vi "Initialize.vi"(11 "Device Reference":T40 format="%.0x") -> (0 "error out":errorcluster, 3 "RT Data":T1 {"Compiled Data"."1.1 APUs"."shared settings"."cycle start" format="%#.15g"; "Compiled Data"."1.0 APUs"."shared settings"."cycle start" format="%#.15g"})   [LabVIEW 2013, in "Engine Simulation Toolkit Engine.lvlib"]
uses:
  Engine Simulation Toolkit Engine.lvlib
  <vilib>/NI Veristand/Custom Device API/Custom Device Item Ref.ctl
  RT Data.ctl
  Shared/Compiled Data.ctl
  Shared/Engine Init Data.ctl
  Shared/1.0 APU Engine Data.ctl
  Shared/1.0 APU Engine FIFO Idxs.ctl
  Shared/Engine Status Data.ctl
  Shared/1.0 Analog Replay Engine Data.ctl
  Shared/1.0 Analog Replay FIFO Idxs.ctl
  Shared/1.0 Digital Pattern Gen Engine Data.ctl
  Shared/1.0 Digital Pattern Gen FIFO Idxs.ctl
  Shared/1.0 Event Timing Capture Engine Data.ctl
  Shared/1.0 Event Timing Capture FIFO Idxs.ctl
  Shared/1.0 Event Timing Measure Engine Data.ctl
  Shared/1.0 Event Timing Measure FIFO Idxs.ctl
  Shared/1.0 Knock Sensor Engine Data.ctl
  Shared/1.0 Knock Sensor FIFO Idxs.ctl
  Shared/1.0 Knock Cylinder Engine Data.ctl
  Shared/1.0 Knock Cylinder FIFO Idxs.ctl
  Shared/1.0 Directional Speed Engine Data.ctl
  Shared/1.0 Directional Speed FIFO Idxs.ctl
  Shared/1.1 APU Engine Data.ctl
  Shared/1.1 Event Timing Measure Engine Data.ctl
  Shared/1.3 Digital Pattern Gen Engine Data.ctl
  Shared/1.3 Digital Pattern Gen FIFO Idxs.ctl
  Shared/Bitfile EST Version.ctl
  Shared/1.3 APU Engine Data.ctl
  FPGA Refs.ctl
  APU 1.0 Run Refs.ctl
  APU 1.0 Output Ref.ctl
  APU 1.0 Input Ref.ctl
  Analog Replay 1.0 Input Ref.ctl
  Digital Pattern Gen 1.0 Input Ref.ctl
  Event Timing Capture 1.0 Output Ref.ctl
  Event Timing Measure 1.0 Output Ref.ctl
  Knock Cylinder 1.0 Input Ref.ctl
  Knock Sensor 1.0 Input Ref.ctl
  Directional Speed 1.0 Input Ref.ctl
  Digital Pattern Gen 1.3 Run Refs.ctl
  Digital Pattern Gen 1.3 Settings Ref.ctl
  Shared/Properties.vi
  <vilib>/NI Veristand/Custom Device API/Get Item Property (Variant).vi
  <vilib>/NI Veristand/Custom Device API/Custom Device API.lvlib
  Shared/Engine Simulation Toolkit Shared.lvlib
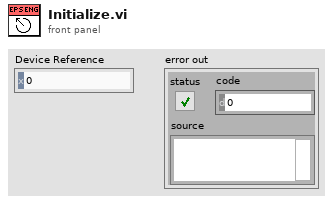
[diagram p1: front panel]
types:
  T1 = typedef "Engine Simulation Toolkit Engine.lvlib/RT Data.ctl" = cluster{"Compiled Data":T2, "FPGA Refs":T27}
  T2 = typedef "Engine Simulation Toolkit Shared.lvlib/Compiled Data.ctl" = cluster{"Init":T3, "1.0 APUs":T4[], "Status":T6, "DevOutFIFO":refnum<k33>, "DevInFIFO":refnum<k33>, "Device Inputs":dbl[], "Device Outputs":dbl[], "Last Device Inputs":dbl[], "1.0 Analog Replays":T7[], "Unused Analog Replays":string[], "1.0 Digital Pattern Gens":T9[], "Unused Digital Pattern Gens":string[], "1.0 Event Captures":T11[], "1.0 Event Measures":T13[], "1.0 Knock Sensors":T15[], "1.0 Knock Cylinders":T17[], "1.0 Directional Speed":T19[], "Unused Directional Sensors":string[], "1.1 APUs":T21[], "1.1 Event Measures":T22[], "1.3 Digital Pattern Gens":T23[], "Bitfile EST Version":T25, "1.3 APUs":T26[]}
  T3 = typedef "Engine Simulation Toolkit Shared.lvlib/Engine Init Data.ctl" = cluster{"CPU":i32, "RIO Address":string, "Decimation":i64, "Priority":i32, "Name":string, "Bitfile Path":path, "Input FIFO Size":i32, "Output FIFO Size":i32}
  T4 = typedef "Engine Simulation Toolkit Shared.lvlib/1.0 APU Engine Data.ctl" = cluster{"register names":cluster{"shared settings":string, "input":string, "settings":string, "output":string}, "shared settings":cluster{"cycle start":fxp<+,2,2>, "crank start":u16, "stuck limit":fxp<+,18,18>}, "settings":cluster{"acceleration":fxp<+,18,-20>, "max cycle":fxp<+,2,2>, "enable accel":bool}, "FIFO indexes":T5, "input":cluster{"desired speed":fxp<+/-,23,2>, "reset":bool}, "degrees of 1 cycle u16":dbl, "degrees of 1 crank u16":dbl}
  T5 = typedef "Engine Simulation Toolkit Shared.lvlib/1.0 APU Engine FIFO Idxs.ctl" = cluster{"inputs":cluster{"desired speed":i32, "reset":i32}, "outputs":cluster{"crank angle":i32, "cycle angle":i32, "actual speed":i32}}
  T6 = typedef "Engine Simulation Toolkit Shared.lvlib/Engine Status Data.ctl" = cluster{"FIFO indexes":cluster{"code":i32, "loop duration":i32, "late count":i32}}
  T7 = typedef "Engine Simulation Toolkit Shared.lvlib/1.0 Analog Replay Engine Data.ctl" = cluster{"register names":cluster{"load input":string, "settings":string, "input":string}, "settings":cluster{"ReverseNegate":bool, "CycleAngle":bool, "SpeedThreshold":fxp<+/-,23,2>, "AOBelowThreshold":i16}, "FIFO indexes":T8, "input":cluster{"Offset":i16, "VScaleSlope":fxp<+,18,6>, "VScaleIntercept":fxp<+/-,18,3>}, "offset convert":dbl, "DAC LUT":i16[], "SE_VScaleIntercept":fxp<+/-,18,3>, "SE_VScaleSlope":fxp<+,18,6>, "VOverride":bool, "ResetVolts":bool}
  T8 = typedef "Engine Simulation Toolkit Shared.lvlib/1.0 Analog Replay FIFO Idxs.ctl" = cluster{"enable voltage":i32, "volt slope":i32, "volt intercept":i32, "offset":i32}
  T9 = typedef "Engine Simulation Toolkit Shared.lvlib/1.0 Digital Pattern Gen Engine Data.ctl" = cluster{"register names":cluster{"load input":string, "settings":string, "input":string}, "settings":cluster{"edge 1":u16, "edge 2":u16, "cycle angle":bool, "enabled":bool, "first falling":bool}, "FIFO indexes":T10, "input":cluster{"Offset":i16}, "offset convert":dbl, "Position LUT":u16[]}
  T10 = typedef "Engine Simulation Toolkit Shared.lvlib/1.0 Digital Pattern Gen FIFO Idxs.ctl" = cluster{"offset":i32}
  T11 = typedef "Engine Simulation Toolkit Shared.lvlib/1.0 Event Timing Capture Engine Data.ctl" = cluster{"register names":cluster{"output":string}, "FIFO indexes":T12, "degrees of 1 u16":dbl, "wrap":bool, "window min":u16, "duration convert":dbl, "default start":dbl, "default end":dbl, "ref angle":dbl}
  T12 = typedef "Engine Simulation Toolkit Shared.lvlib/1.0 Event Timing Capture FIFO Idxs.ctl" = cluster{"start angle":i32, "end angle":i32, "duration":i32}
  T13 = typedef "Engine Simulation Toolkit Shared.lvlib/1.0 Event Timing Measure Engine Data.ctl" = cluster{"register names":cluster{"settings":string, "output":string}, "settings":cluster{"max":u16, "min":u16, "active high":bool, "wrap":bool, "full window":bool}, "FIFO indexes":T14}
  T14 = typedef "Engine Simulation Toolkit Shared.lvlib/1.0 Event Timing Measure FIFO Idxs.ctl" = cluster{"stuck active":i32, "win all active":i32, "win orph start":i32, "win orph end":i32}
  T15 = typedef "Engine Simulation Toolkit Shared.lvlib/1.0 Knock Sensor Engine Data.ctl" = cluster{"register names":cluster{"settings":string, "input":string}, "settings":cluster{"low freq (periods/tick)":fxp<+,32,0>, "high freq (periods/tick)":fxp<+,32,0>, "duration (1.25MHz tics)":fxp<+,18,18>, "low freq speed slope":fxp<+,16,-3>, "low freq speed intercept":fxp<+,10,-10>, "low freq by speed":bool}, "DAC multiplier":dbl, "FIFO indexes":T16, "input":cluster{"low freq scaler":fxp<+,10,0>}}
  T16 = typedef "Engine Simulation Toolkit Shared.lvlib/1.0 Knock Sensor FIFO Idxs.ctl" = cluster{"amp":i32}
  T17 = typedef "Engine Simulation Toolkit Shared.lvlib/1.0 Knock Cylinder Engine Data.ctl" = cluster{"register names":cluster{"settings":string, "input":string}, "settings":cluster{"seed":u16, "reset":bool}, "input":cluster{"probability compare":u16, "high freq scaler":fxp<+,10,0>, "trigger position":u16}, "DAC multiplier":dbl, "FIFO indexes":T18, "Angle multiplier":dbl}
  T18 = typedef "Engine Simulation Toolkit Shared.lvlib/1.0 Knock Cylinder FIFO Idxs.ctl" = cluster{"prob":i32, "amp":i32, "pos":i32}
  T19 = typedef "Engine Simulation Toolkit Shared.lvlib/1.0 Directional Speed Engine Data.ctl" = cluster{"register names":cluster{"settings":string, "input":string, "load input":string}, "settings":cluster{"Upper Value":u16, "Lower Value":u16, "Upper Index":fxp<+,10,10>, "Lower Index":fxp<+,10,10>, "Enabled":bool}, "input":cluster{"td (tics)":u16, "tf (tics)":u16, "tr (tics)":u16}, "FIFO indexes":T20, "Tooth Centers LUT":u16[]}
  T20 = typedef "Engine Simulation Toolkit Shared.lvlib/1.0 Directional Speed FIFO Idxs.ctl" = cluster{"td":i32, "tf":i32, "tr":i32}
  T21 = typedef "Engine Simulation Toolkit Shared.lvlib/1.1 APU Engine Data.ctl" = cluster{"register names":cluster{"shared settings":string, "input":string, "settings":string, "output":string, "go":string}, "shared settings":cluster{"cycle start":fxp<+,2,2>, "crank start":u16, "stuck limit":fxp<+,18,18>}, "settings":cluster{"acceleration":fxp<+,18,-20>, "max cycle":fxp<+,2,2>, "enable accel":bool}, "FIFO indexes":T5, "input":cluster{"desired speed":fxp<+/-,23,2>, "reset":bool}, "degrees of 1 cycle u16":dbl, "degrees of 1 crank u16":dbl}
  T22 = typedef "Engine Simulation Toolkit Shared.lvlib/1.1 Event Timing Measure Engine Data.ctl" = cluster{"register names":cluster{"settings":string, "output":string}, "settings":cluster{"max":u16, "min":u16, "active high":bool, "wrap":bool}, "FIFO indexes":T14}
  T23 = typedef "Engine Simulation Toolkit Shared.lvlib/1.3 Digital Pattern Gen Engine Data.ctl" = cluster{"register names":cluster{"load input":string, "settings":string, "input":string}, "settings":cluster{"edge 1":u16, "edge 2":u16, "cycle angle":bool, "enabled":bool, "first falling":bool, "fault":bool, "fault wrap":bool, "fault value":bool, "fault count":fxp<+,4,4>, "use fault count":bool}, "FIFO indexes":T24, "input":cluster{"Offset":i16}, "deg to u16 scale":dbl, "Position LUT":u16[], "# of teeth":i16, "max angle":dbl}
  T24 = typedef "Engine Simulation Toolkit Shared.lvlib/1.3 Digital Pattern Gen FIFO Idxs.ctl" = cluster{"offset":i32, "command":i32, "rotations":i32, "start angle":i32, "stop angle":i32, "tooth to rem":i32, "trigger":i32, "valid":i32}
  T25 = typedef "Engine Simulation Toolkit Shared.lvlib/Bitfile EST Version.ctl" = enum16{"1.0", "1.1", "1.2", "1.3"}
  T26 = typedef "Engine Simulation Toolkit Shared.lvlib/1.3 APU Engine Data.ctl" = cluster{"register names":cluster{"shared settings":string, "input":string, "settings":string, "output":string, "go":string}, "shared settings":cluster{"start":fxp<+,17,17>, "stuck limit":fxp<+,18,18>}, "settings":cluster{"acceleration":fxp<+,18,-20>, "enable accel":bool}, "FIFO indexes":T5, "input":cluster{"desired speed":fxp<+/-,23,2>, "reset":bool}, "degrees of 1 cycle u16":dbl, "degrees of 1 crank u16":dbl}
  T27 = typedef "Engine Simulation Toolkit Engine.lvlib/FPGA Refs.ctl" = cluster{"1.0 APUs":T28[], "FPGA ref":refnum<k20>, "1.0 Analog Replays":T31[], "1.0 Dig Pat Gens":T32[], "1.0 Event Captures":T33[], "1.0 Event Measures":T34[], "1.0 Knock Cylinders":T35[], "1.0 Knock Sensors":T36[], "1.0 Directional Speed Sensors":T37[], "1.3 Dig Pat Gens":T38[]}
  T28 = typedef "Engine Simulation Toolkit Engine.lvlib/APU 1.0 Run Refs.ctl" = cluster{"output reference":T29, "input reference":T30}
  T29 = typedef "Engine Simulation Toolkit Engine.lvlib/APU 1.0 Output Ref.ctl" = refnum<k20>
  T30 = typedef "Engine Simulation Toolkit Engine.lvlib/APU 1.0 Input Ref.ctl" = refnum<k20>
  T31 = typedef "Engine Simulation Toolkit Engine.lvlib/Analog Replay 1.0 Input Ref.ctl" = refnum<k20>
  T32 = typedef "Engine Simulation Toolkit Engine.lvlib/Digital Pattern Gen 1.0 Input Ref.ctl" = refnum<k20>
  T33 = typedef "Engine Simulation Toolkit Engine.lvlib/Event Timing Capture 1.0 Output Ref.ctl" = refnum<k20>
  T34 = typedef "Engine Simulation Toolkit Engine.lvlib/Event Timing Measure 1.0 Output Ref.ctl" = refnum<k20>
  T35 = typedef "Engine Simulation Toolkit Engine.lvlib/Knock Cylinder 1.0 Input Ref.ctl" = refnum<k20>
  T36 = typedef "Engine Simulation Toolkit Engine.lvlib/Knock Sensor 1.0 Input Ref.ctl" = refnum<k20>
  T37 = typedef "Engine Simulation Toolkit Engine.lvlib/Directional Speed 1.0 Input Ref.ctl" = refnum<k20>
  T38 = typedef "Engine Simulation Toolkit Engine.lvlib/Digital Pattern Gen 1.3 Run Refs.ctl" = cluster{"input":T32, "settings":T39}
  T39 = typedef "Engine Simulation Toolkit Engine.lvlib/Digital Pattern Gen 1.3 Settings Ref.ctl" = refnum<k20>
  T40 = typedef "Custom Device API.lvlib/Custom Device Item Ref.ctl" = u64
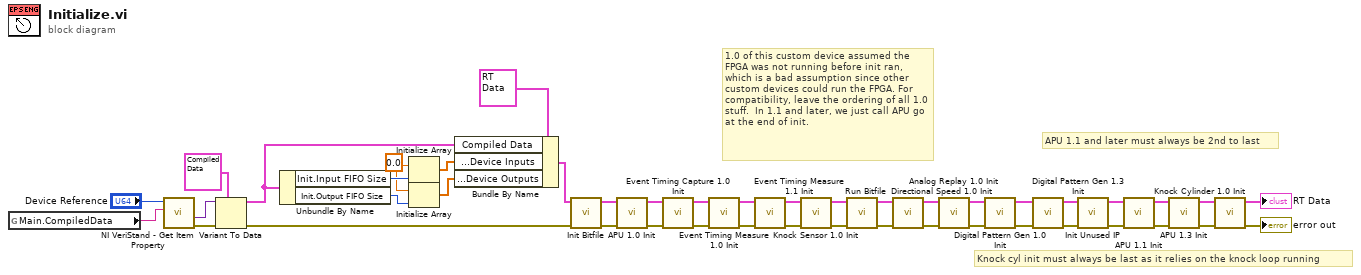
[diagram p0: block diagram]
diagram:
  w31 = 0.0
  # "Knock cyl init must always be last as it relies on the knock loop running"
  # "APU 1.1 and later must always be 2nd to last"
  # "1.0 of this custom device assumed the FPGA was not running before init ran, which is a bad assumption since other custom devices could run the FPGA. For compatibility, leave the ordering of all 1.0 stuff.  In 1.1 and later, we just call APU go at the end of init."
  n1 = global read "Properties.vi" "Main.CompiledData"() -> (w44:string)
  n2 = call-poly <vilib>:"NI VeriStand - Get Item Property.vi"("Property Name"=w44, "Item Ref in"="Device Reference") -> ("error out"=w40:errorcluster, "Value"=w43:variant)  [unwired: 6 in, 2 out]
  n3 = Variant To Data(error in=w40, type=T2 {"Init"={"CPU"=0, "RIO Address"="", "Decimation"=0, "Priority"=0, "Name"="", "Bitfile Path"=path "", "Input FIFO Size"=0, "Output FIFO Size"=0}, "1.0 APUs"=[], "Status"={"FIFO indexes"={"code"=0, "loop duration"=0, "late count"=0}}, "DevOutFIFO"=refnum, "DevInFIFO"=refnum, "Device Inputs"=[], "Device Outputs"=[], "Last Device Inputs"=[], "1.0 Analog Replays"=[], "Unused Analog Replays"=[], "1.0 Digital Pattern Gens"=[], "Unused Digital Pattern Gens"=[], "1.0 Event Captures"=[], "1.0 Event Measures"=[], "1.0 Knock Sensors"=[], "1.0 Knock Cylinders"=[], "1.0 Directional Speed"=[], "Unused Directional Sensors"=[], "1.1 APUs"=[], "1.1 Event Measures"=[], "1.3 Digital Pattern Gens"=[], "Bitfile EST Version"=enum."1.0", "1.3 APUs"=[]} ("Compiled Data"), Variant=w43) -> (data=w34:T2, error out=w39:errorcluster)
  n4 = Unbundle By Name(w34) -> ("Init.Input FIFO Size"=w33:i32, "Init.Output FIFO Size"=w30:i32)
  n5 = Initialize Array(w31, w33) -> (w32:dbl[])
  n6 = Initialize Array(w31, w30) -> (w29:dbl[])
  n7 = Bundle By Name(cluster=T1 {"Compiled Data"={"Init"={"CPU"=0, "RIO Address"="", "Decimation"=0, "Priority"=0, "Name"="", "Bitfile Path"=path "", "Input FIFO Size"=0, "Output FIFO Size"=0}, "1.0 APUs"=[], "Status"={"FIFO indexes"={"code"=0, "loop duration"=0, "late count"=0}}, "DevOutFIFO"=refnum, "DevInFIFO"=refnum, "Device Inputs"=[], "Device Outputs"=[], "Last Device Inputs"=[], "1.0 Analog Replays"=[], "Unused Analog Replays"=[], "1.0 Digital Pattern Gens"=[], "Unused Digital Pattern Gens"=[], "1.0 Event Captures"=[], "1.0 Event Measures"=[], "1.0 Knock Sensors"=[], "1.0 Knock Cylinders"=[], "1.0 Directional Speed"=[], "Unused Directional Sensors"=[], "1.1 APUs"=[], "1.1 Event Measures"=[], "1.3 Digital Pattern Gens"=[], "Bitfile EST Version"=enum."1.0", "1.3 APUs"=[]}, "FPGA Refs"={"1.0 APUs"=[], "FPGA ref"=refnum, "1.0 Analog Replays"=[], "1.0 Dig Pat Gens"=[], "1.0 Event Captures"=[], "1.0 Event Measures"=[], "1.0 Knock Cylinders"=[], "1.0 Knock Sensors"=[], "1.0 Directional Speed Sensors"=[], "1.3 Dig Pat Gens"=[]}} ("RT Data"), "Compiled Data"=w34, "Compiled Data.Device Inputs"=w32, "Compiled Data.Device Outputs"=w29) -> (w35:T1)
  n8 = call "Init Bitfile.vi"("error in (no error)"=w39, "rt Data in"=w35) -> ("error out"=w38:errorcluster, "rt Data out"=w36:T1)  [unwired: 8 in]
  n9 = call "APU 1.0 Init.vi"("error in (no error)"=w38, "rt Data in"=w36) -> ("error out"=w37:errorcluster, "rt Data out"=w24:T1)  [unwired: 8 in]
  n10 = call "Event Timing Capture 1.0 Init.vi"("error in (no error)"=w37, "rt Data in"=w24) -> ("error out"=w25:errorcluster, "rt Data out"=w22:T1)  [unwired: 8 in]
  n11 = call "Event Timing Measure 1.0 Init.vi"("error in (no error)"=w25, "rt Data in"=w22) -> ("error out"=w23:errorcluster, "rt Data out"=w21:T1)  [unwired: 8 in]
  n12 = call "Event Timing Measure 1.1 Init.vi"("error in (no error)"=w23, "rt Data in"=w21) -> ("error out"=w20:errorcluster, "rt Data out"=w11:T1)  [unwired: 8 in]
  n13 = call "Knock Sensor 1.0 Init.vi"("error in (no error)"=w20, "rt Data in"=w11) -> ("error out"=w12:errorcluster, "rt Data out"=w10:T1)  [unwired: 8 in]
  n14 = call "Run Bitfile.vi"("error in (no error)"=w12, "rt data in"=w10) -> ("error out"=w19:errorcluster, "rt data out"=w18:T1)  [unwired: 8 in]
  n15 = call "Directional Speed 1.0 Init.vi"("error in (no error)"=w19, "rt Data in"=w18) -> ("error out"=w14:errorcluster, "rt Data out"=w13:T1)  [unwired: 8 in]
  n16 = call "Analog Replay 1.0 Init.vi"("error in (no error)"=w14, "rt Data in"=w13) -> ("error out"=w27:errorcluster, "rt Data out"=w26:T1)  [unwired: 8 in]
  n17 = call "Digital Pattern Gen 1.0 Init.vi"("error in (no error)"=w27, "rt Data in"=w26) -> ("error out"=w9:errorcluster, "rt Data out"=w7:T1)  [unwired: 8 in]
  n18 = call "Digital Pattern Gen 1.3 Init.vi"("error in (no error)"=w9, "rt Data in"=w7) -> ("error out"=w8:errorcluster, "rt Data out"=w2:T1)  [unwired: 8 in]
  n19 = call "Init Unused IP.vi"("error in (no error)"=w8, "rt data in"=w2) -> ("error out"=w3:errorcluster, "rt data out"=w1:T1)  [unwired: 8 in]
  n20 = call "APU 1.1 Init.vi"("error in (no error)"=w3, "rt Data in"=w1) -> ("error out"=w17:errorcluster, "rt Data out"=w5:T1)  [unwired: 8 in]
  n21 = call "APU 1.3 Init.vi"("error in (no error)"=w17, "rt Data in"=w5) -> ("error out"=w6:errorcluster, "rt Data out"=w4:T1)  [unwired: 8 in]
  n22 = call "Knock Cylinder 1.0 Init.vi"("error in (no error)"=w6, "rt Data in"=w4) -> ("error out"=→"error out":errorcluster, "rt Data out"=→"RT Data":T1)  [unwired: 8 in]
